vi "WLC for dsDNA + ssDNA_YCC.vi"() -> ()   [LabVIEW 2014]
uses:
  <vilib>/Utility/file.llb/Read From Spreadsheet File (DBL).vi
  <vilib>/gmath/NumericalOptimization/Nonlinear Curve Fit LM formula string.vi
  <vilib>/Utility/file.llb/Write To Spreadsheet File (DBL).vi
  <vilib>/gmath/NI_Gmath.lvlib
panel:
  out "deltaL":dbl
  out "output cluster":T1
  out "dsDNA bp for folded (bp)":dbl
  out "ssDNA nt for folded (nt)":dbl
  out "ssDNA nt for unfolded (nt)":dbl
  out "U-Force":dbl[](array[numeric])
  out "best nonlinear fit for unfolded Extension":dbl[](array[numeric])
  out "best nonlinear fit for folded Extension":dbl[](array[numeric])
  in  "Save?":bool
  in  "stop":bool
  in  "file path (dialog if empty)":path=path "D:/YCC/20190429/204118-F+U-2500.00-1.00 um s^-1-L-4.69 nm avg step-20R-h300-1-1-raw-U-ForecExtension Only.txt"
  out "fitting result for ssDNA difference (nt)":dbl=50.71744125895441
  out "F-Force":dbl[](array[numeric])
  out "Ex":dbl[](array[numeric])
  in  "unfold+fold?":bool
  out "Force-unfold 2":dbl[](array[numeric])
  out "Force-fold 2":dbl[](array[numeric])
  out "Ex-unfold 2":dbl[](array[numeric])
  out "Ex-fold 2":dbl[](array[numeric])
  out "Force-unfold":dbl[](array[numeric])
  out "Force-fold":dbl[](array[numeric])
  out "Ex-fold":dbl[](array[numeric])
  out "Ex-unfold":dbl[](array[numeric])
  in  "Tab Control":T2(tab)
  out "XY Graph":cluster{"all rows":dbl[], "all rows":dbl[]}(graph)
  out "XY Graph 2":cluster{"all rows":dbl[], "all rows":dbl[]}(graph)
  out "XY Graph 4":cluster{dbl[], dbl[]}[](graph)
  out "XY Graph 5":cluster{dbl[], dbl[]}(graph)
  out "XY Graph 6":cluster{"best nonlinear fit":dbl[], dbl[]}[](graph)
  out "best fit for folded state":dbl[](array[numeric])
  in  "upper bound force for folded":dbl=13.0
  in  "upper bound extension for folded":dbl=1130.0
  in  "lower bound force for folded":dbl=5.0
  out "XY Graph 7":cluster{"best nonlinear fit":dbl[], dbl[]}[](graph)
  out "best fit for unfolded state":dbl[](array[numeric])
  in  "lower bound force for unfolded":dbl=15.0
  out "XY Graph 8":cluster{"best nonlinear fit":dbl[], dbl[]}[](graph)=[{"best nonlinear fit"=[1038.0330205673613, 1043.7185958577572, 1044.1558684196555, 1050.2879988681962, 1060.4769691999934, 1059.3948179811991, 1057.853565828751, 1065.7984103563997, 1068.6846982155607, 1073.5602269385115, 1081.329695723092, 1080.8999575243838, 1079.3566661683478, 1085.2841590404873, 1092.96058737889, 1095.351763882275, 1100.4870949911547, 1099.7187986528597, 1106.5727869521195, 1107.5315414752133, 1107.6484559404782, 1113.0033704274604, 1116.591376928688, 1118.931801904476, 1121.34241994843, 1123.498297961807, 1126.5922820000274], [3.18708, 3.438821, 3.459056, 3.756871, 4.31567, 4.252169, 4.163513, 4.643798, 4.833528, 5.174651, 5.778643, 5.7431, 5.617617, 6.118648, 6.852835, 7.104214, 7.686007, 7.595086, 8.459938, 8.591251, 8.607451, 9.395877, 9.979663, 10.387151, 10.830652, 11.249051, 11.887912]}, {"best nonlinear fit"=[1159.0281066256528, 1161.5383333271998, 1162.3420637225367, 1165.2070788539822, 1166.8942422456175, 1168.3817194289143, 1169.850482087464, 1172.3994604578224, 1175.1650893927117, 1176.9909665840107, 1180.4998831628072, 1181.3689998592602, 1181.4538313079074, 1184.4681180394457, 1187.597096720695, 1188.9029244725086, 1190.5981171382134, 1192.7638108589474, 1195.2134847506977, 1196.530378246371, 1198.6238213224515, 1200.7221633450886, 1201.4148464356078, 1204.3918686742195, 1204.9590230454778, 1207.8301999339246, 1208.2336005079694], [14.574345, 15.218147, 15.431821, 16.224345, 16.714266, 17.160926, 17.615808, 18.438683, 19.380799, 20.031607, 21.348153, 21.687821, 21.721266, 22.943465, 24.282182, 24.862055, 25.633439, 26.649425, 27.839633, 28.497302, 29.568184, 30.672468, 31.043707, 32.67645, 32.994258, 34.635529, 34.870396]}, {"best nonlinear fit"=[638.728515, 642.246514, 643.683915, 648.61245, 652.706031, 659.782953, 664.273021, 663.134065, 665.444288, 672.345125, 676.22682, 678.322951, 684.571212, 685.050727, 692.06957, 696.040883, 697.446469, 701.641829, 709.09346, 710.446962, 716.872475, 721.395099, 725.440954, 727.787064, 731.393119, 734.200197, 734.151081, 741.511798, 745.072067, 751.348447, 753.203026, 756.099836, 762.798137, 763.683227, 768.323146, 774.033714, 778.03341, 782.36623, 783.935842, 790.786664, 795.169854, 797.683737, 802.138184, 807.329326, 811.069937, 816.093668, 819.684173, 820.215093, 827.713093, 832.397494, 835.431831, 840.388569, 844.025948, 850.206783, 852.823721, 858.713513, 865.013047, 866.217067, 869.768889, 871.343862, 877.247965, 884.61154, 888.488266, 890.657001, 895.260505, 901.06674, 903.571381, 907.268997, 912.176826, 918.530635, 921.603537, 924.244857, 931.280393, 932.783652, 938.648998, 942.236254, 945.970031, 951.692839, 956.291816, 960.165498, 965.199998, 970.219539, 972.949146, 976.225472, 983.398173, 985.606724, 990.660298, 994.236104, 1000.496151, 1003.653259, 1008.605635, 1011.846346, 1017.520309, 1020.220686, 1022.793798, 1027.157761, 1032.646259, 1035.507184, 1039.044046, 1045.917144, 1048.355556, 1051.714035, 1053.906481, 1058.924963, 1064.061011, 1066.648797, 1070.553531, 1073.794208, 1075.883635, 1080.82176, 1086.161418, 1088.746638, 1090.330254, 1094.045848, 1096.336229, 1101.561134, 1102.659857, 1106.942647, 1111.72696, 1113.212685, 1115.596631, 1118.747825, 1121.760818, 1124.894413, 1127.116838, 1129.734511, 1131.792882, 1139.771893, 1144.495385, 1150.300745, 1151.328493, 1153.52261, 1155.507019, 1157.84731, 1161.955495, 1163.723685, 1166.736551, 1169.937301, 1173.117477, 1174.838425, 1176.107585, 1178.557912, 1178.396872, 1182.113568, 1187.041212, 1187.320023, 1187.18035, 1190.016746, 1192.127145, 1193.31516, 1193.86154, 1196.468865, 1197.520102, 1198.470728, 1202.211794, 1201.218293, 1205.186385, 1204.222739, 1208.523286], [0.326492, 0.348509, 0.705544, 0.507954, 0.445812, 0.095332, 0.219138, 0.572777, 0.811076, 0.301109, 0.286389, 0.568499, 0.167664, 0.724765, 0.197622, 0.179122, 0.593621, 0.543207, 0.055582, 0.377824, 0.046477, 0.146491, 0.163366, 0.113898, 0.178112, 0.383412, 1.090171, 0.508794, 0.592131, 0.200817, 0.588631, 0.797057, 0.333508, 0.90529, 0.811154, 0.526273, 0.549709, 0.515149, 0.983624, 0.495968, 0.457723, 0.763478, 0.716668, 0.535726, 0.62377, 0.476317, 0.596499, 1.291629, 0.686155, 0.608327, 0.843051, 0.717368, 0.843197, 0.487441, 0.81176, 0.51305, 0.136063, 0.739518, 0.89524, 1.438014, 1.141953, 0.56138, 0.661771, 1.100129, 1.06305, 0.789723, 1.171072, 1.319246, 1.228291, 0.849192, 1.127868, 1.497101, 0.982338, 1.587056, 1.310293, 1.49801, 1.658511, 1.413444, 1.399727, 1.537041, 1.436587, 1.340231, 1.721082, 1.991828, 1.449978, 1.948311, 1.852163, 2.068977, 1.72016, 2.02945, 1.959776, 2.256598, 2.035442, 2.453, 2.902205, 2.967995, 2.791559, 3.18708, 3.438821, 2.963119, 3.459056, 3.756871, 4.31567, 4.252169, 4.163513, 4.643798, 4.833528, 5.174651, 5.778643, 5.7431, 5.617617, 6.118648, 6.852835, 7.104214, 7.686007, 7.595086, 8.459938, 8.591251, 8.607451, 9.395877, 9.979663, 10.387151, 10.830652, 11.249051, 11.887912, 12.437116, 13.124861, 12.392508, 12.442613, 12.232991, 13.178986, 13.848605, 14.574345, 15.218147, 15.431821, 16.224345, 16.714266, 17.160926, 17.615808, 18.438683, 19.380799, 20.031607, 21.348153, 21.687821, 21.721266, 22.943465, 24.282182, 24.862055, 25.633439, 26.649425, 27.839633, 28.497302, 29.568184, 30.672468, 31.043707, 32.67645, 32.994258, 34.635529, 34.870396]}]
  in  "Ex offset":dbl=600.0
  in  "Force offset":dbl=35.0
  out "Extension":dbl[](array[numeric])
  out "Force":dbl[](array[numeric])
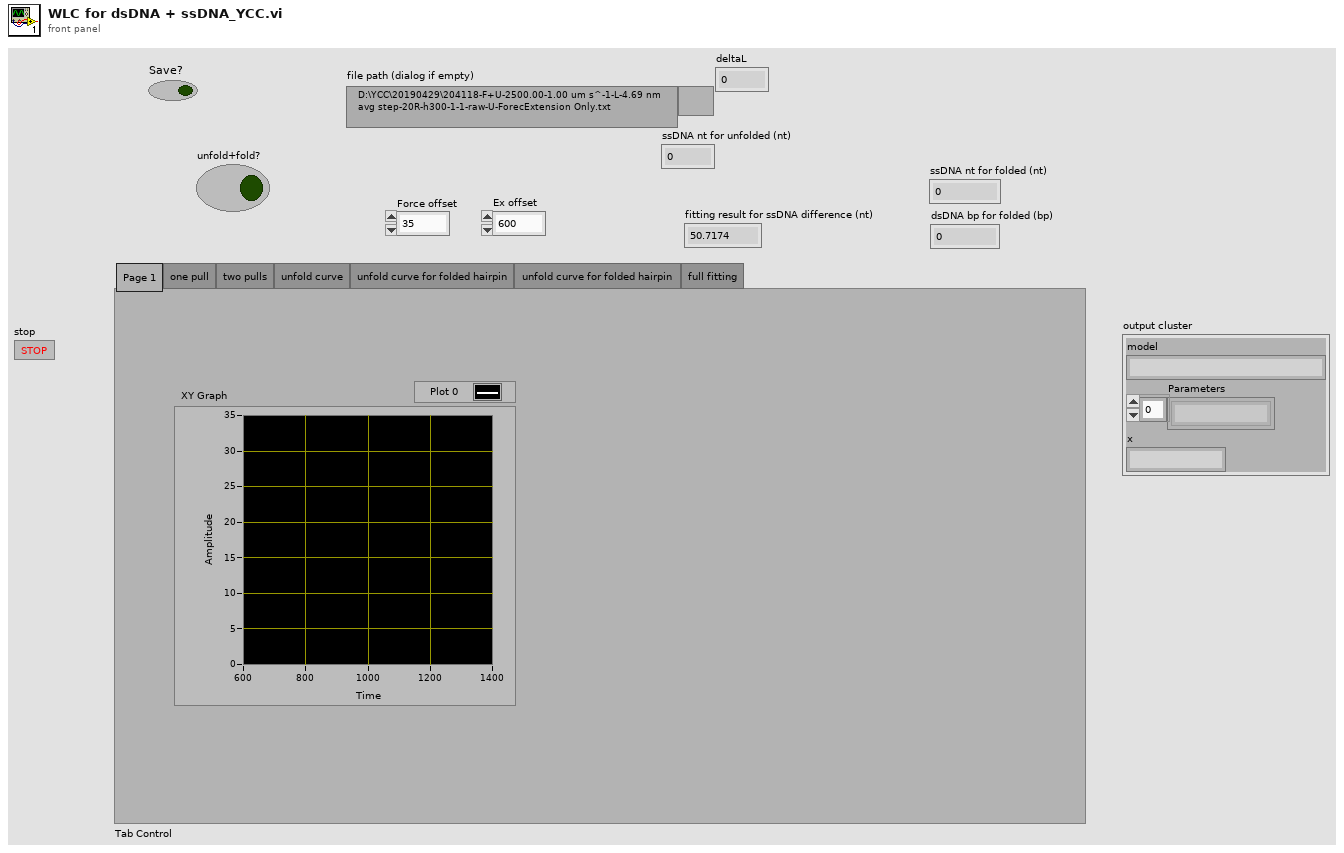
[diagram p1: front panel]
types:
  T1 = cluster{"model":string, "Parameters":string[], "x":string}
  T2 = enum32{"Page 1", "one pull", "two pulls", "unfold curve", "unfold curve for folded hairpin", "unfold curve for folded hairpin ", "full fitting"}
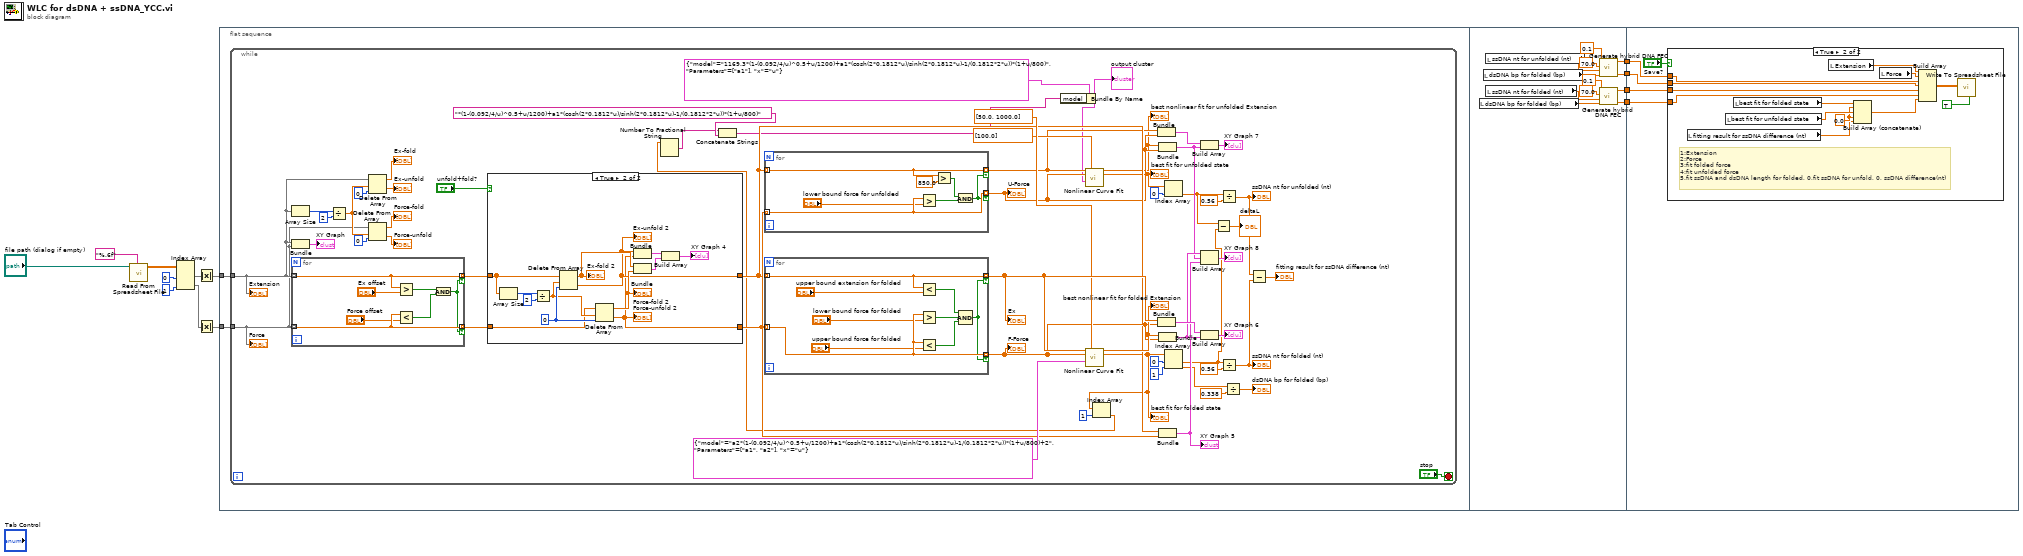
[diagram p0: block diagram]
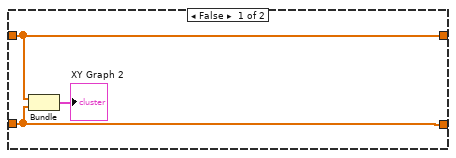
[diagram p2: hidden frame]
diagram:
  n1 = call-poly <vilib>:"Read From Spreadsheet File.vi"("format (%.3f)"="%.6f", "file path (dialog if empty)"="file path (dialog if empty)") -> ("all rows"=w13:dbl[][])  [unwired: 5 in, 4 out]
  n2 = Index Array(array=w13, index (col) #1=0 ("disabled index (col)"), index (col) #2=1 ("index (col)")) -> (element #1=w8:dbl[], element #2=w7:dbl[])  [unwired: 2 in]
  n3 = Absolute Value(x=w8) -> (abs(x)=w5:dbl[])
  n4 = Absolute Value(x=w7) -> (abs(x)=w6:dbl[])
  n5 = flat-sequence {
    tunnel: w6 -> [w15]
    tunnel: w5 -> [w14]
    tunnel: [w119] -> w4
    tunnel: [w118] -> w3
    tunnel: [w117] -> w2
    tunnel: [w116] -> w1
    tunnel: w4 -> [w128]
    tunnel: w3 -> [w127]
    tunnel: w2 -> [w126]
    tunnel: w1 -> [w125]
    frame #0 {
      n6 = while {
        tunnel: w14 -> [w72]
        tunnel: w15 -> [w41]
        stop <- "stop" stop-if-true
        n7 = Array Size(array=w72) -> (size(s)=w71:i32)
        n8 = Bundle(w72, w41) -> (→"XY Graph":cluster{dbl[], dbl[]})  [unwired: 1 in]
        n9 = for {
          tunnel: w41 -> [w112] mode=indexing
          tunnel: [w112] -> w61 mode=indexing if=w106
          tunnel: w72 -> [w110] mode=indexing
          tunnel: [w110] -> w62 mode=indexing if=w106
          n10 = Greater?(x=w110, y="Ex offset") -> (0:w108:bool)
          n11 = Less?(x=w112, y="Force offset") -> (x < y?=w107:bool)
          n12 = And(x=w108, y=w107) -> (x .and. y?=w106:bool)
        }
        n13 = Divide(x=w71, y=2) -> (x/y=w66:dbl)
        n14 = Delete From Array(array=w72, length=w66, index=0) -> (deleted portion=→"Ex-unfold":dbl[], array with subset deleted=→"Ex-fold":dbl[])
        n15 = Delete From Array(array=w41, length=w66, index=0) -> (deleted portion=→"Force-unfold":dbl[], array with subset deleted=→"Force-fold":dbl[])
        n16 = case shown="True" "unfold+fold?" {
          tunnel: w62 -> [w91 w103]
          tunnel: w61 -> [w90 w100]
          tunnel: [w91 w94] -> w53
          tunnel: [w90 w93] -> w54
          frame False {
            n17 = Bundle(w91, w90) -> (→"XY Graph 2":cluster{dbl[], dbl[]})  [unwired: 1 in]
          }
          frame True {
            w102 = 0 ("index")
            n18 = Array Size(array=w103) -> (size(s)=w105:i32)
            n19 = Divide(x=w105, y=2) -> (x/y=w101:dbl)
            n20 = Delete From Array(array=w103, length=w101, index=w102) -> (deleted portion=w94:dbl[], array with subset deleted=w99:dbl[])
            "Ex-fold 2" <- w99
            "Ex-unfold 2" <- w94
            n21 = Delete From Array(array=w100, length=w101, index=w102) -> (deleted portion=w93:dbl[], array with subset deleted=w98:dbl[])
            "Force-fold 2" <- w98
            "Force-unfold 2" <- w93
            n22 = Bundle(w94, w93) -> (w97:cluster{dbl[], dbl[]})  [unwired: 1 in]
            n23 = Bundle(w99, w98) -> (w96:cluster{dbl[], dbl[]})  [unwired: 1 in]
            n24 = Build Array(w97, w96) -> (→"XY Graph 4":cluster{dbl[], dbl[]}[])
          }
        }
        n25 = for {
          tunnel: w54 -> [w80] mode=indexing
          tunnel: [w80] -> w51 mode=indexing if=w76
          tunnel: w53 -> [w79] mode=indexing
          tunnel: [w79] -> w50 mode=indexing if=w76
          n26 = Greater?(x=w80, y="lower bound force for unfolded") -> (0:w77:bool)
          n27 = Greater?(x=w79, y=850.0) -> (0:w78:bool)
          n28 = And(x=w78, y=w77) -> (x .and. y?=w76:bool)
        }
        "U-Force" <- w51
        n29 = for {
          tunnel: w54 -> [w89] mode=indexing
          tunnel: [w89] -> w55 mode=indexing if=w84
          tunnel: w53 -> [w88] mode=indexing
          tunnel: [w88] -> w59 mode=indexing if=w84
          n30 = Less?(x=w88, y="upper bound extension for folded") -> (x < y?=w87:bool)
          n31 = Greater?(x=w89, y="lower bound force for folded") -> (0:w86:bool)
          n32 = Less?(x=w89, y="upper bound force for folded") -> (x < y?=w85:bool)
          n33 = Compound Arithmetic op=AND(w87, w86, w85) -> (w84:bool)
        }
        "Ex" <- w59
        "F-Force" <- w55
        n34 = call-poly <vilib>:"Nonlinear Curve Fit.vi"("Y"=w59, "initial parameters"=dbl[] [50.0, 1000.0], "X"=w55, "model description"=T1 {"model"="a2*(1-(0.092/4/u)^0.5+u/1200)+a1*(cosh(2*0.1812*u)/sinh(2*0.1812*u)-1/(0.1812*2*u))*(1+u/800)+2", "Parameters"=["a1", "a2"], "x"="u"}) -> ("best nonlinear fit"=w56:dbl[], "best fit parameters"=w25:dbl[])  [unwired: 3 in, 7 out]
        "best fit for folded state" <- w25
        "best nonlinear fit for folded Extension" <- w56
        n35 = Index Array(array=w25, index=1) -> (element=w23:dbl)
        n36 = Number To Fractional String(number=w23) -> (F-format string=w22:string)  [unwired: 3 in]
        n37 = Concatenate Strings(w22, "*(1-(0.092/4/u)^0.5+u/1200)+a1*(cosh(2*0.1812*u)/sinh(2*0.1812*u)-1/(0.1812*2*u))*(1+u/800)" ("model")) -> (w21:string)
        n38 = Bundle By Name(cluster=T1 {"model"="1169.3*(1-(0.092/4/u)^0.5+u/1200)+a1*(cosh(2*0.1812*u)/sinh(2*0.1812*u)-1/(0.1812*2*u))*(1+u/800)", "Parameters"=["a1"], "x"="u"} ("model description"), "model"=w21) -> (w20:T1)
        "output cluster" <- w20
        n39 = call-poly <vilib>:"Nonlinear Curve Fit.vi"("Y"=w50, "initial parameters"=dbl[] [100.0], "X"=w51, "model description"=w20) -> ("best nonlinear fit"=w40:dbl[], "best fit parameters"=w36:dbl[])  [unwired: 3 in, 7 out]
        "best fit for unfolded state" <- w36
        "best nonlinear fit for unfolded Extension" <- w40
        n40 = Bundle(w50, w51) -> (w45:cluster{dbl[], dbl[]})  [unwired: 1 in]
        n41 = Bundle(w59, w55) -> (w47:cluster{dbl[], dbl[]})  [unwired: 1 in]
        n42 = Bundle("best nonlinear fit"=w40, w51) -> (w19:cluster{"best nonlinear fit":dbl[], dbl[]})  [unwired: 1 in]
        n43 = Bundle("best nonlinear fit"=w56, w55) -> (w46:cluster{"best nonlinear fit":dbl[], dbl[]})  [unwired: 1 in]
        n44 = Bundle(w53, w54) -> (w43:cluster{dbl[], dbl[]})  [unwired: 1 in]
        "XY Graph 5" <- w43
        n45 = Index Array(array=w36, index=0) -> (element=w17:dbl)
        n46 = Index Array(array=w25, index #1=0 ("index"), index #2=1 ("index")) -> (element #1=w18:dbl, element #2=w29:dbl)
        n47 = Build Array(w45, w19) -> (→"XY Graph 7":cluster{"best nonlinear fit":dbl[], dbl[]}[])
        n48 = Build Array(w46, w19, w43) -> (→"XY Graph 8":cluster{"best nonlinear fit":dbl[], dbl[]}[])
        n49 = Build Array(w47, w46) -> (→"XY Graph 6":cluster{"best nonlinear fit":dbl[], dbl[]}[])
        n50 = Subtract(x=w17, y=w18) -> (x-y=→"deltaL":dbl)
        n51 = Divide(x=w17, y=0.56 ("Numeric")) -> (x/y=w32:dbl)
        "ssDNA nt for unfolded (nt)" <- w32
        n52 = Divide(x=w18, y=0.56 ("Numeric")) -> (x/y=w31:dbl)
        "ssDNA nt for folded (nt)" <- w31
        n53 = Divide(x=w29, y=0.338 ("Numeric")) -> (x/y=→"dsDNA bp for folded (bp)":dbl)
        n54 = Subtract(x=w32, y=w31) -> (x-y=→"fitting result for ssDNA difference (nt)":dbl)
        "Force" <- w41
        "Extension" <- w72
      }
    }
    frame #1 {
      n55 = local read "dsDNA bp for folded (bp)"() -> (w115:dbl)
      n56 = local read "dsDNA bp for folded (bp)"() -> (w123:dbl)
      n57 = local read "ssDNA nt for unfolded (nt)"() -> (w124:dbl)
      n58 = local read "ssDNA nt for folded (nt)"() -> (w122:dbl)
      n59 = call "Generate hybrid DNA FEC.vi"("dF (pN)"=0.1 ("Start Force (pN)"), "End Force (pN)"=70.0, "ssDNA Length (nt)"=w124, "dsDNA Length (bp)"=w123) -> ("Extension array (nm)"=w119:dbl[], "Force Array (pN)"=w118:dbl[])  [unwired: 1 in, 2 out]
      n60 = call "Generate hybrid DNA FEC.vi"("dF (pN)"=0.1 ("Start Force (pN)"), "End Force (pN)"=70.0, "ssDNA Length (nt)"=w122, "dsDNA Length (bp)"=w115) -> ("Extension array (nm)"=w117:dbl[], "Force Array (pN)"=w116:dbl[])  [unwired: 1 in, 2 out]
    }
    frame #2 {
      n61 = case shown="True" "Save?" {
        tunnel: w128 -> [_ w133]
        tunnel: w127 -> [_ w132]
        tunnel: w126 -> [_ w131]
        tunnel: w125 -> [_ w130]
        frame False {
        }
        frame True {
          w138 = 0.0
          # "1:Extension\n2:Force\n3:fit folded force\n4:fit unfolded force\n5.fit ssDNA and dsDNA length for folded, 0,fit ssDNA for unfold, 0, ssDNA difference(nt)"
          n62 = local read "fitting result for ssDNA difference (nt)"() -> (w137:dbl)
          n63 = local read "best fit for unfolded state"() -> (w139:dbl[])
          n64 = local read "best fit for folded state"() -> (w140:dbl[])
          n65 = local read "Extension"() -> (w142:dbl[])
          n66 = Build Array (concatenate)(w140, w138, w139, w138, w137) -> (w134:dbl[])
          n67 = local read "Force"() -> (w141:dbl[])
          n68 = Build Array(w142, w141, w133, w132, w131, w130, w134) -> (w136:dbl[][])
          n69 = call-poly <vilib>:"Write To Spreadsheet File.vi"("transpose? (no:F)"=TRUE, "2D data"=w136) -> ()  [unwired: 6 in, 1 out]
        }
      }
    }
  }
